vi "Channel Array to Channel List String.vi"(10 "Channel Array":T1(array[cluster])) -> (2 "Channel List String":string)   [LabVIEW 2018, in "Keithley 7001.lvlib"]
uses:
  <instrlib>/Keithley 7001/Keithley 7001.lvlib
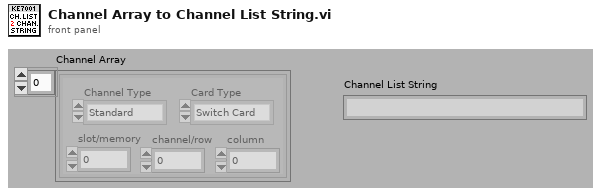
[diagram p1: front panel]
types:
  T1 = cluster{"slot/memory":i32, "channel/row":i32, "column":i32, "Channel Type":enum16{"Standard", "Memory"}, "Card Type":enum16{"Switch Card", "Matrix Card"}}[]
  T2 = cluster{"slot/memory":i32, "channel/row":i32, "column":i32, "Channel Type":enum16{"Standard", "Memory"}, "Card Type":enum16{"Switch Card", "Matrix Card"}}
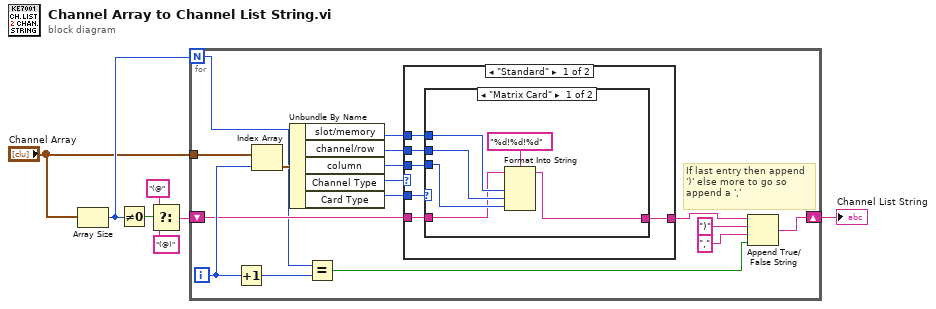
[diagram p0: block diagram]
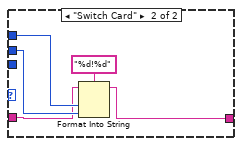
[diagram p2: hidden frame]
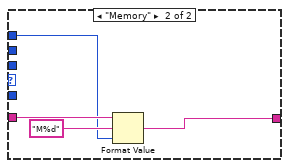
[diagram p3: hidden frame]
diagram:
  n1 = Array Size(array="Channel Array") -> (size(s)=w6:i32)
  n2 = Not Equal To 0?(x=w6) -> (x != 0?=w4:bool)
  n3 = Select(t="(@", s=w4, f="(@)") -> (s? t:f=w5:string)
  n4 = for {
    N: w6 -> [w8]
    tunnel: "Channel Array" -> [w23]
    shift-right: [w10] -> w7
    shift-left: w5 -> [w19]
    i -> [w22]
    # "If last entry then append\n')' else more to go so\nappend a ','"
    n5 = Increment(x=w22) -> (x+1=w9:i32)
    n6 = Index Array(array=w23, index=w22) -> (element=w21:T2)
    n7 = Unbundle By Name(w21) -> ("slot/memory"=w18:i32, "channel/row"=w16:i32, "column"=w15:i32, "Channel Type"=w20:enum16{"Standard", "Memory"}, "Card Type"=w17:enum16{"Switch Card", "Matrix Card"})
    n8 = Equal?(x=w8, y=w9) -> (x = y?=w13:bool)
    n9 = case shown="\"Standard\"" w20 {
      tunnel: w19 -> [w28 w43]
      tunnel: w18 -> [w27 w42]
      tunnel: [w24 w41] -> w14
      tunnel: w17 -> [w29 _]
      tunnel: w16 -> [w26 _]
      tunnel: w15 -> [w25 _]
      frame "Standard" {
        n10 = case shown="\"Matrix Card\"" w29 {
          tunnel: w28 -> [w30 w36]
          tunnel: w27 -> [w34 w39]
          tunnel: w26 -> [w33 w38]
          tunnel: [w31 w37] -> w24
          tunnel: w25 -> [w32 _]
          frame "Matrix Card" {
            n11 = Format Into String(format string="%d!%d!%d", initial string=w30, w34, w33, w32) -> (resulting string=w31:string)  [unwired: 1 in, 1 out]
          }
          frame "Switch Card" {
            n12 = Format Into String(format string="%d!%d", initial string=w36, w39, w38) -> (resulting string=w37:string)  [unwired: 1 in, 1 out]
          }
        }
      }
      frame "Memory" {
        n13 = Format Value(string ("")=w43, format string="M%d", value (0)=w42) -> (output string=w41:string)
      }
    }
    n14 = Append True/False String(1:w13, 2:",", 3:")", 4:w14) -> (0:w10:string)
  }
  "Channel List String" <- w7
